vi "Script Find current Constants.vi"(8 "error in":errorcluster, 11 "Selction Owning Folder":path) -> (0 "error out":errorcluster, 1 "All Constant VIS":path[](array[path]), 2 "Constants Info":T1[](array[typedef]))   [LabVIEW 2020, in "ConstantErrorsMaker.lvlib"]
uses:
  ConstantErrorsMaker.lvlib
  Constant Info--cluster.ctl
  <vilib>/Utility/traverseref.llb/TRef TravTarget.ctl
  <vilib>/Utility/traverseref.llb/VI Scripting - Traverse.lvlib
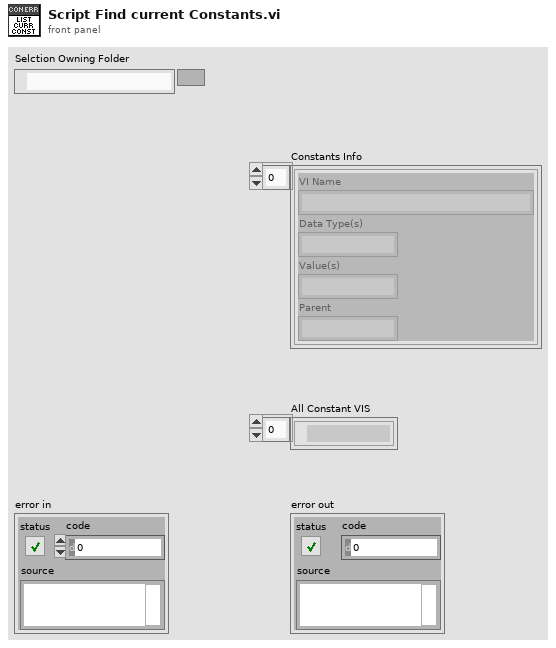
[diagram p1: front panel]
types:
  T1 = typedef "ConstantErrorsMaker.lvlib/Constant Info--cluster.ctl" = cluster{"VI Name":string, "Data Type(s)":string, "Value(s)":string, "Parent":string}
  T2 = typedef "TRef TravTarget.ctl" = enum16{"FP", "BD", "Other"}
  T3 = typedef "NI_Data Type.lvlib/Data Type.ctl" = enum8{"Invalid Type", "Void", "I8", "I16", "I32", "I64", "U8", "U16", "U32", "U64", "Single Float", "Double Float", "Extended Float", "Single Complex", "Double Complex", "Extended Complex", "Enum U8", "Enum U16", "Enum U32", "Enum U64", "Single Float With Unit", "Double Float With Unit", "Extended Float With Unit", "Single Complex with Unit", "Double Complex with Unit", "Extended Complex with Unit", "Boolean", "String", "Path", "Picture", "Tag", "Array", "Cluster", "Variant", "LV Variant", "Waveform", "Timestamp", "Digital Waveform", "Digital Data", "ExpressData", "Refnum", "External Data", "VI", "Poly VI", "LabVIEW Class Instance", "Fixed Point", "Set Collection", "Map Collection"}
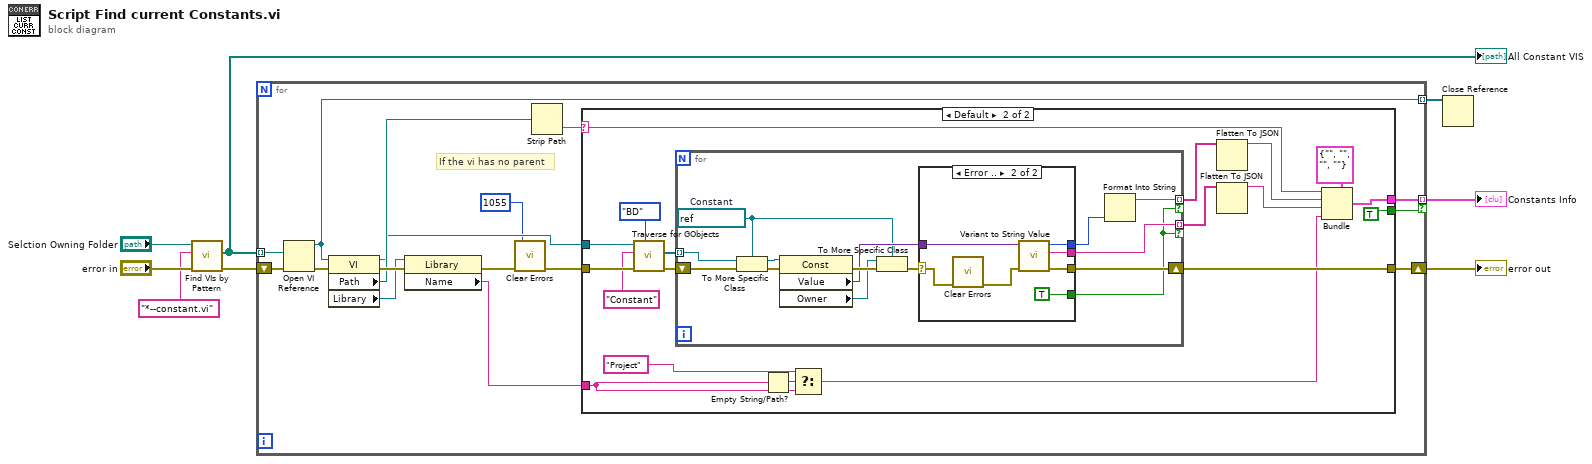
[diagram p0: block diagram]
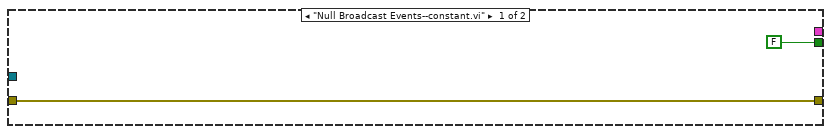
[diagram p2: hidden frame]
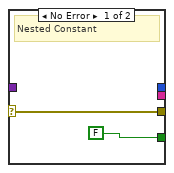
[diagram p3: hidden frame]
diagram:
  n1 = call "Find VIs by Pattern.vi"("error in"="error in", "pattern"="*--constant.vi", "Selction Owning Folder"="Selction Owning Folder") -> ("error out"=w6:errorcluster, "All Files in Dir"=w4:path[])  [unwired: 7 in]
  "All Constant VIS" <- w4
  n2 = for {
    tunnel: w4 -> [w18] mode=indexing
    shift-right: [w22] -> w7
    shift-left: w6 -> [w21]
    tunnel: [w14] -> w2 mode=indexing if=w12
    tunnel: [w13] -> w3 mode=indexing
    # "If the vi has no parent"
    n3 = Open VI Reference(vi path=w18, error in (no error)=w21) -> (vi reference=w13:refnum<vi>, error out=w23:errorcluster)  [unwired: 4 in]
    n4 = property class="VI"(reference=w13, error in=w23) -> (reference out=w15:refnum<vi>, error out=w24:errorcluster, "Path"=w16:path, "Library"=w11:refnum<vi>)
    n5 = property class="Library"(reference=w11, error in=w24) -> (error out=w20:errorcluster, "Name"=w9:string)  [unwired: 1 out]
    n6 = call <vilib>:"Clear Errors.vi"("error in (no error)"=w20, "specific error code to clear (0: all)"=1055) -> ("error out"=w19:errorcluster)  [unwired: 4 in, 1 out]
    n7 = Strip Path(path=w16) -> (name=w17:string)  [unwired: 1 out]
    n8 = case shown="Default" w17 {
      selector: w17 -> [_ w42]
      tunnel: w19 -> [w26 w45]
      tunnel: [w26 w43] -> w22
      tunnel: w15 -> [_ w41]
      tunnel: [_ w37] -> w14
      tunnel: [FALSE TRUE] -> w12
      tunnel: w9 -> [_ w28]
      frame "Null Broadcast Events--constant.vi" {
      }
      frame Default {
        n9 = call <vilib>:"Traverse for GObjects.vi"("Traverse Target"=TRef_TravTarget."BD", "error in (no error)"=w45, "Class Name"="Constant", "VI Refnum"=w41) -> ("error out"=w44:errorcluster, "References"=w40:refnum<vi>[])  [unwired: 4 in, 2 out]
        n10 = for {
          shift-right: [w57] -> w43
          shift-left: w44 -> [w59]
          tunnel: w40 -> [w54] mode=indexing
          tunnel: [w51] -> w33 mode=indexing if=w48
          tunnel: [w47] -> w34 mode=indexing if=w48
          w49 = refnum<vi> refnum  # Constant
          n11 = To More Specific Class(target class=w49, reference=w54, error in=w59) -> (specific class reference=w53:refnum<vi>, error out=w58:errorcluster)
          n12 = property class="Const"(reference=w53, error in=w58) -> (error out=w56:errorcluster, "Value"=w52:variant, "Owner"=w50:refnum<vi>)  [unwired: 1 out]
          n13 = To More Specific Class(target class=w49, reference=w50, error in=w56) -> (error out=w55:errorcluster)  [unwired: 1 out]
          n14 = case shown="Error .." w55 {
            selector: w55 -> [w61 w68]
            tunnel: [w61 w66] -> w57
            tunnel: w52 -> [_ w64]
            tunnel: [_ w62] -> w51
            tunnel: [_ w63] -> w46
            tunnel: [FALSE TRUE] -> w48
            frame No Error {
              # "Nested Constant"
            }
            frame Error {
              n15 = call <vilib>:"Clear Errors.vi"("error in (no error)"=w68) -> ("error out"=w67:errorcluster)  [unwired: 5 in, 1 out]
              n16 = call "Variant to String Value.vi"("error in"=w67, "Value"=w64) -> ("error out"=w66:errorcluster, "String"=w62:string, "type"=w63:T3)  [unwired: 7 in]
            }
          }
          n17 = Format Into String(w46) -> (resulting string=w47:string)  [unwired: 3 in, 1 out]
        }
        n18 = Empty String/Path?(string/path=w28) -> (empty?=w30:bool)
        n19 = Select(t="Project", s=w30, f=w28) -> (s? t:f=w27:string)
        n20 = Flatten To JSON(anything=w34) -> (JSON string=w32:string)  [unwired: 2 in, 1 out]
        n21 = Flatten To JSON(anything=w33) -> (JSON string=w31:string)  [unwired: 2 in, 1 out]
        n22 = Bundle(cluster=T1 {"VI Name"="", "Data Type(s)"="", "Value(s)"="", "Parent"=""} ("output cluster"), "VI Name"=w42, "Data Type(s)"=w32, "Value(s)"=w31, "Parent"=w27) -> (w37:T1)
      }
    }
  }
  "error out" <- w7
  "Constants Info" <- w2
  n23 = Close Reference(reference=w3) -> ()  [unwired: 1 in, 1 out]
